vi "core_is_code_plus_eco.vi"(4 "code":i32) -> (1 "has + ECO?":bool)   [LabVIEW 2015]
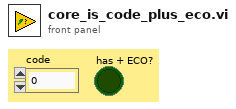
[diagram p1: front panel]
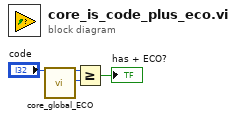
[diagram p0: block diagram]
diagram:
  n1 = call "core_global_ECO.vi"() -> ("LVutils global ECO"=w1:i32)
  n2 = Greater Or Equal?(x="code", y=w1) -> (x >= y?=→"has + ECO?":bool)
